vi "deactivateHWUserLED.vi"(8 "error in (no error)":errorcluster, 11 "CompactRIO in":refnum<class "CompactRIO.lvclass">) -> (0 "error out":errorcluster, 3 "CompactRIO out":refnum<class "CompactRIO.lvclass">)   [LabVIEW 2012, in "CompactRIO.lvclass"]
uses:
  CompactRIO.lvclass
  <vilib>/NI_Real-Time Target Support.lvlib
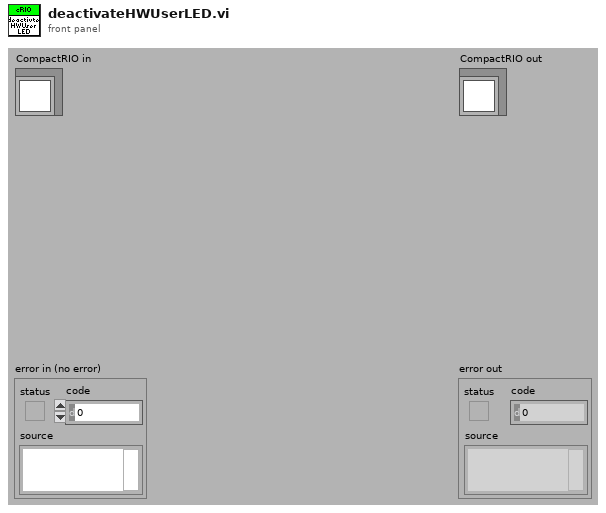
[diagram p1: front panel]
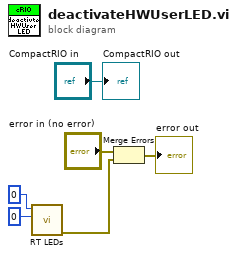
[diagram p0: block diagram]
diagram:
  n1 = call <vilib>:"RT LEDs.vi"("State"=0, "LED Num"=0 ("State")) -> ("error out"=w2:errorcluster)  [unwired: 4 in, 1 out]
  n2 = Merge Errors("error in (no error)", w2) -> (→"error out":errorcluster)
  "CompactRIO out" <- "CompactRIO in"
